vi "Process.vi"(8 "error in":errorcluster, 11 "lia host in":refnum<class "LIA Host Interface RT.lvclass">) -> (0 "error out":errorcluster, 3 "lia host out":refnum<class "LIA Host Interface RT.lvclass">)   [LabVIEW 2017, in "LIA Host Interface RT.lvclass"]
uses:
  LIA Host Interface RT.lvclass
  Properties/StopProcess_GET.vi
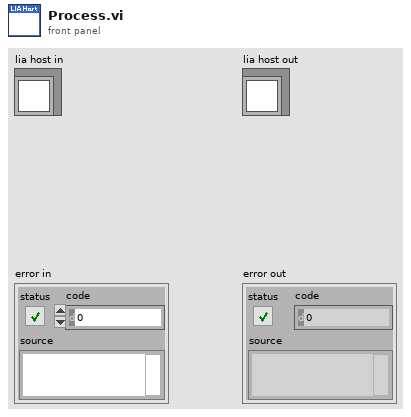
[diagram p1: front panel]
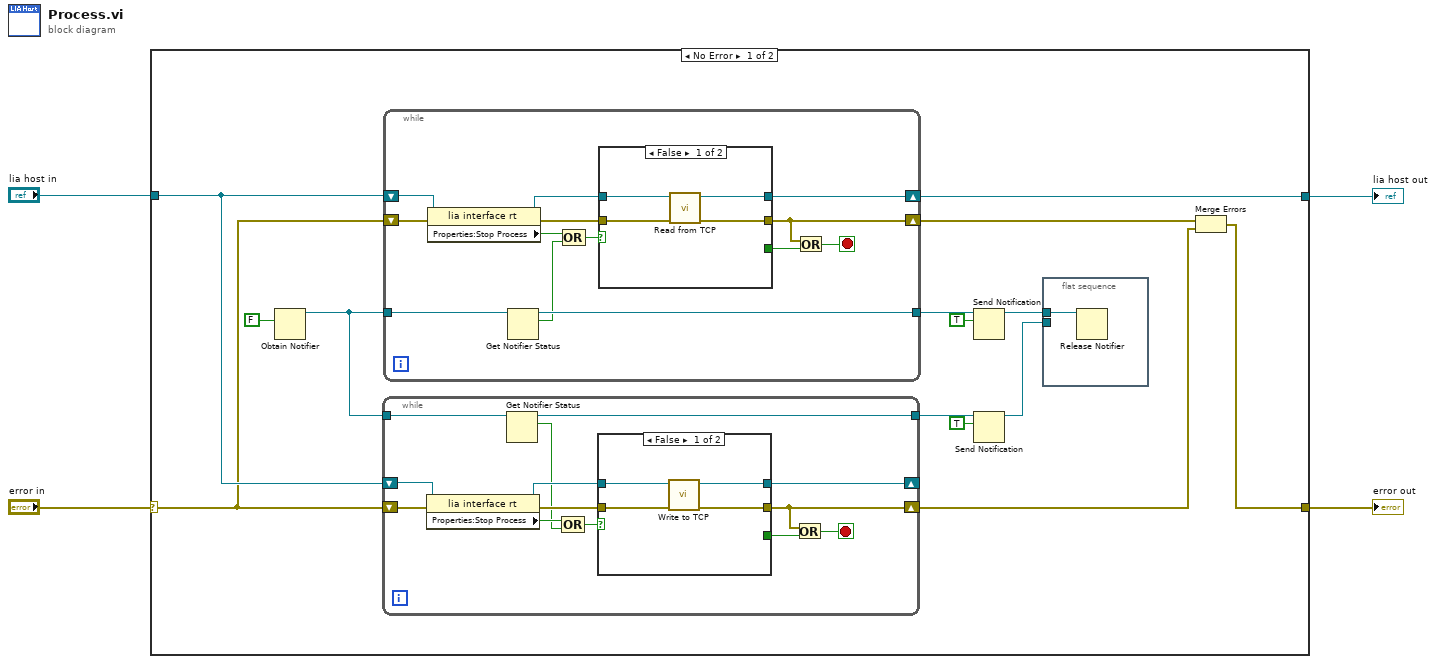
[diagram p0: block diagram]
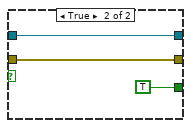
[diagram p2: hidden frame]
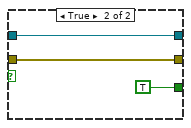
[diagram p3: hidden frame]
diagram:
  n1 = case shown="No Error" "error in" {
    selector: "error in" -> [w5 w60]
    tunnel: "lia host in" -> [w15 w61]
    tunnel: [w9 w61] -> w3
    tunnel: [w6 w60] -> w2
    frame No Error {
      n2 = Obtain Notifier(notification data type=FALSE) -> (notifier out=w14:refnum<notifier>)  [unwired: 3 in, 2 out]
      n3 = while {
        shift-right: [w27] -> w8
        shift-left: w5 -> [w29]
        shift-right: [w28] -> _
        shift-left: w15 -> [w32]
        tunnel: w14 -> [w23]
        tunnel: [w24] -> w12
        stop <- w26 stop-if-true
        n4 = property class="lia interface rt"(reference=w32, error in=w29) -> (reference out=w31:refnum<class "LIA Host Interface RT.lvclass">, error out=w30:errorcluster, "Properties:Stop Process"=w22:bool)
        n5 = Get Notifier Status(notifier=w23) -> (notifier out=w24:refnum<notifier>, current notification=w21:bool)  [unwired: 1 in, 3 out]
        n6 = Compound Arithmetic op=OR(w22, w21) -> (w20:bool)
        n7 = case shown="False" w20 {
          tunnel: w31 -> [w36 w39]
          tunnel: w30 -> [w35 w38]
          tunnel: [w34 w38] -> w27
          tunnel: [w33 w39] -> w28
          tunnel: [_ TRUE] -> w25
          frame False {
            n8 = call "Write to TCP.vi"("error in"=w35, "lia interface in"=w36) -> ("error out"=w34:errorcluster, "lia interface out"=w33:refnum<class "LIA Host Interface RT.lvclass">)  [unwired: 8 in]
          }
          frame True {
          }
        }
        n9 = Or(x=w27, y=w25) -> (x .or. y?=w26:bool)
      }
      n10 = while {
        shift-right: [w47] -> w7
        shift-left: w5 -> [w49]
        shift-right: [w48] -> w9
        shift-left: w15 -> [w52]
        tunnel: w14 -> [w43]
        tunnel: [w44] -> w17
        stop <- w46 stop-if-true
        n11 = property class="lia interface rt"(reference=w52, error in=w49) -> (reference out=w51:refnum<class "LIA Host Interface RT.lvclass">, error out=w50:errorcluster, "Properties:Stop Process"=w42:bool)
        n12 = Get Notifier Status(notifier=w43) -> (notifier out=w44:refnum<notifier>, current notification=w41:bool)  [unwired: 1 in, 3 out]
        n13 = Compound Arithmetic op=OR(w42, w41) -> (w40:bool)
        n14 = case shown="False" w40 {
          tunnel: w51 -> [w56 w59]
          tunnel: w50 -> [w55 w58]
          tunnel: [w54 w58] -> w47
          tunnel: [w53 w59] -> w48
          tunnel: [_ TRUE] -> w45
          frame False {
            n15 = call "Read from TCP.vi"("error in"=w55, "lia host in"=w56) -> ("error out"=w54:errorcluster, "lia host out"=w53:refnum<class "LIA Host Interface RT.lvclass">)  [unwired: 8 in]
          }
          frame True {
          }
        }
        n16 = Or(x=w47, y=w45) -> (x .or. y?=w46:bool)
      }
      n17 = Send Notification(notification=TRUE, notifier=w17) -> (notifier out=w11:refnum<notifier>)  [unwired: 1 in, 1 out]
      n18 = Send Notification(notification=TRUE, notifier=w12) -> (notifier out=w10:refnum<notifier>)  [unwired: 1 in, 1 out]
      n19 = flat-sequence {
        tunnel: w11 -> [w19]
        tunnel: w10 -> [_]
        frame #0 {
          n20 = Release Notifier(notifier=w19) -> ()  [unwired: 2 in, 3 out]
        }
      }
      n21 = Merge Errors(w7, w8) -> (w6:errorcluster)
    }
    frame Error {
    }
  }
  "error out" <- w2
  "lia host out" <- w3
